vi "quack.vi"(8 "error in (no error)":errorcluster, 11 "RubberDuck in":refnum<class "RubberDuck.lvclass">) -> (0 "error out":errorcluster, 2 "State":string, 3 "RubberDuck out":refnum<class "RubberDuck.lvclass">)   [LabVIEW 2013, in "RubberDuck.lvclass"]
uses:
  RubberDuck.lvclass
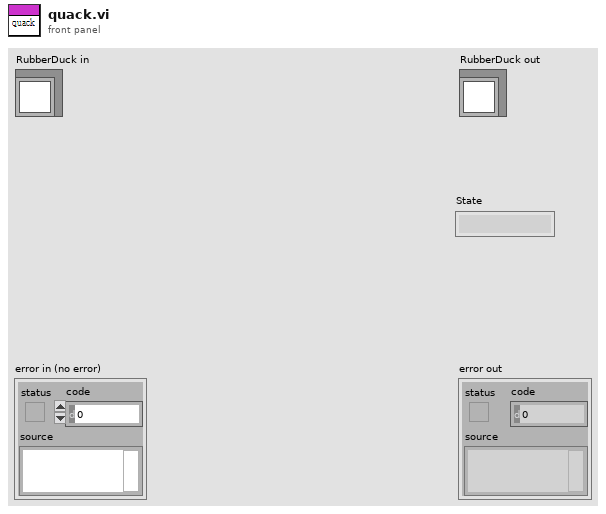
[diagram p1: front panel]
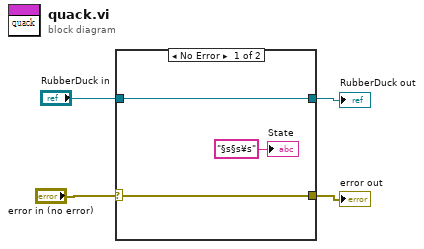
[diagram p0: block diagram]
diagram:
  n1 = case shown="No Error" "error in (no error)" {
    selector: "error in (no error)" -> [w6 w8]
    tunnel: [w7 w9] -> w4
    tunnel: "RubberDuck in" -> [w7 w9]
    tunnel: [w6 w8] -> w1
    frame No Error {
      "State" <- "§s§s¥s" ("State")
    }
    frame Error {
    }
  }
  "error out" <- w1
  "RubberDuck out" <- w4
